vi "Move and get readings--GUI.vi"(4 "OCS ID mod":i32, 6 "DAQ ID mod":i32, 7 "Read sensor?":bool, 8 "error in (no error)":errorcluster, 10 "current position in":dbl, 11 "Motor params":T1) -> (0 "error out":errorcluster, 2 "current position out":dbl caption="Posición actual" format="%0.4f mm", 3 "Sensor reading":dbl)   [LabVIEW 2020, in "GUI.lvlib"]
uses:
  GUI.lvlib
  Support/Motor parameters.ctl
  FGV states.ctl
  NI DAQ/NI DAQ.lvlib
  TDS1002 Oscilloscope/TDS1002 Oscilloscope.lvlib
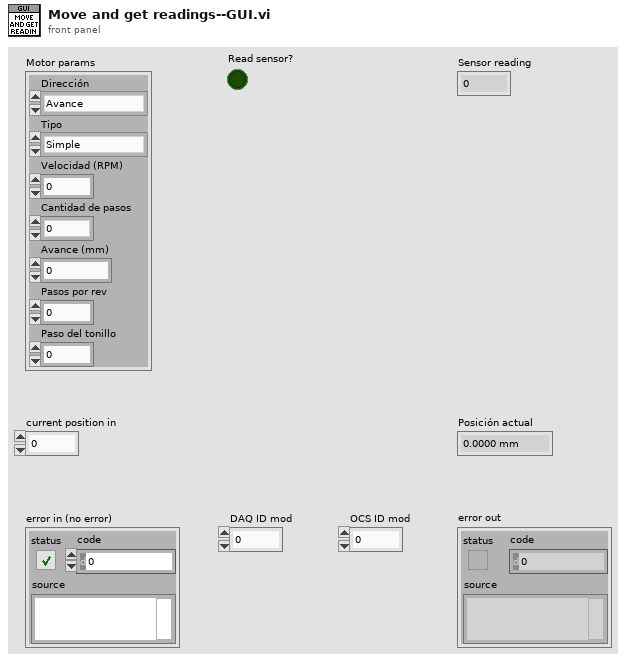
[diagram p1: front panel]
types:
  T1 = typedef "GUI.lvlib/Motor parameters.ctl" = cluster{"Dirección":enum16{"Avance", "Retroceso"}, "Tipo":enum16{"Simple", "Medio paso"}, "Velocidad (RPM)":dbl, "Cantidad de pasos":i32, "Avance (mm)":dbl, "Pasos por rev":dbl, "Paso del tonillo":dbl}
  T2 = typedef "GUI.lvlib/FGV states.ctl" = enum16{"Read", "Full step", "Half step", "Release", "Reset"}
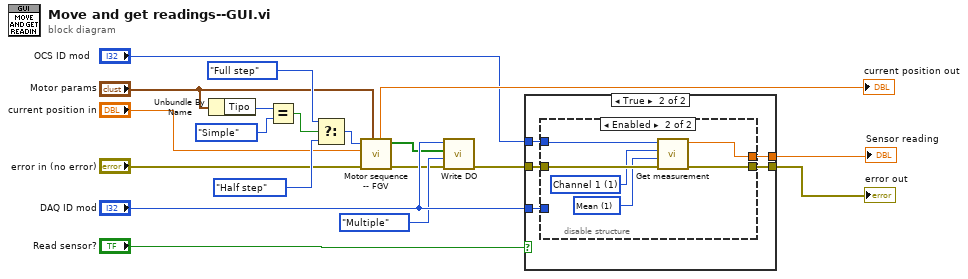
[diagram p0: block diagram]
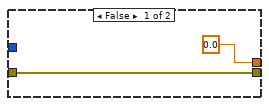
[diagram p2: hidden frame]
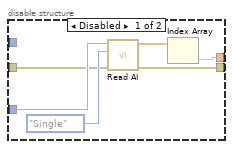
[diagram p3: hidden frame]
diagram:
  n1 = Unbundle By Name("Motor params") -> ("Tipo"=w12:enum16{"Simple", "Medio paso"})
  n2 = Equal?(x=w12, y=enum16{"Simple", "Medio paso"}."Simple") -> (x = y?=w16:bool)
  n3 = Select(t=FGV_states."Full step" ("Action"), s=w16, f=FGV_states."Half step") -> (s? t:f=w17:T2)
  n4 = call "Motor sequence -- FGV.vi"("Motor params"="Motor params", "error in (no error)"="error in (no error)", "current position (in)"="current position in", "Action"=w17) -> ("error out"=w6:errorcluster, "Data out"=w5:bool[], "current position (out)"=→"current position out":dbl)  [unwired: 5 in]
  n5 = call "Write DO.vi"("error in"=w6, "Samples"=enum16{"Single", "Multiple"}."Multiple", "Data"=w5, "Module ID"="DAQ ID mod") -> ("error out"=w18:errorcluster)  [unwired: 7 in]
  n6 = case shown="True" "Read sensor?" {
    tunnel: "DAQ ID mod" -> [_ w26]
    tunnel: w18 -> [w21 w25]
    tunnel: [w21 w24] -> w4
    tunnel: [0.0 ("Value") w23] -> w2
    tunnel: "OCS ID mod" -> [_ w22]
    frame False {
    }
    frame True {
      n7 = disable-structure shown="Enabled" {
        disable-tunnel: w26 -> [w31 _]
        disable-tunnel: w25 -> [w30 w38]
        disable-tunnel: [w29 w37] -> w24
        disable-tunnel: [w27 w36] -> w23
        disable-tunnel: w22 -> [_ w33]
        frame Disabled {
          n8 = call "Read AI.vi"("error in"=w30, "Samples"=enum16{"Single", "Multiple"}."Single", "Module ID"=w31) -> ("error out"=w29:errorcluster, "Data"=w28:dbl[])  [unwired: 6 in, 1 out]
          n9 = Index Array(array=w28) -> (element=w27:dbl)  [unwired: 1 in]
        }
        frame Enabled {
          w34 = 1 items=["Frequency", "Mean", "Period", "Pulse Duty", "Peak to Peak", "Cycle RMS", "Minimum", "Maximum", "Rise Time", "Fall Time", "Positive Width", "Negative Width", "Amplitude", "Cycle Mean", "High", "Low", "Negative Duty", "Positive Overshoot", "Negative Overshoot", "Cursor Mean", "Burst Width", "Positive Pulse Count", "Negative Pulse Count", "Rising Edge Count", "Falling Edge Count", "Area", "Cycle Area", "RMS", "Cursor RMS"] ("Measurement Type")
          w35 = 1 items=["Channel 1"=1, "Channel 2"=2, "Channel 3"=3, "Channel 4"=4] ("Channel")
          n10 = call "Get measurement.vi"("error in"=w38, "Measurement Type"=w34, "Channel"=w35, "Module ID"=w33) -> ("error out"=w37:errorcluster, "Value"=w36:dbl)  [unwired: 5 in, 1 out]
        }
      }
    }
  }
  "Sensor reading" <- w2
  "error out" <- w4
